vi "single path processing time test.vi"() -> ()   [LabVIEW 2010]
panel:
  out "x-y":u16
  out "updated max path lengths":u16[](array[numeric])
  in  "index":i32
  in  "Wheel Angle":i8
  in  "y LIDAR position(in)":i16
  in  "x LIDAR position(in)":i16
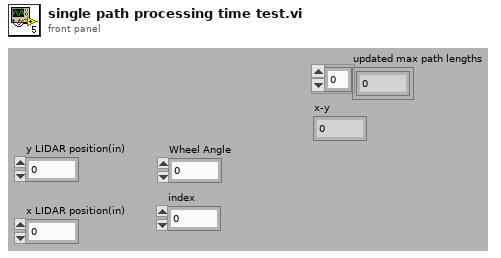
[diagram p1: front panel]
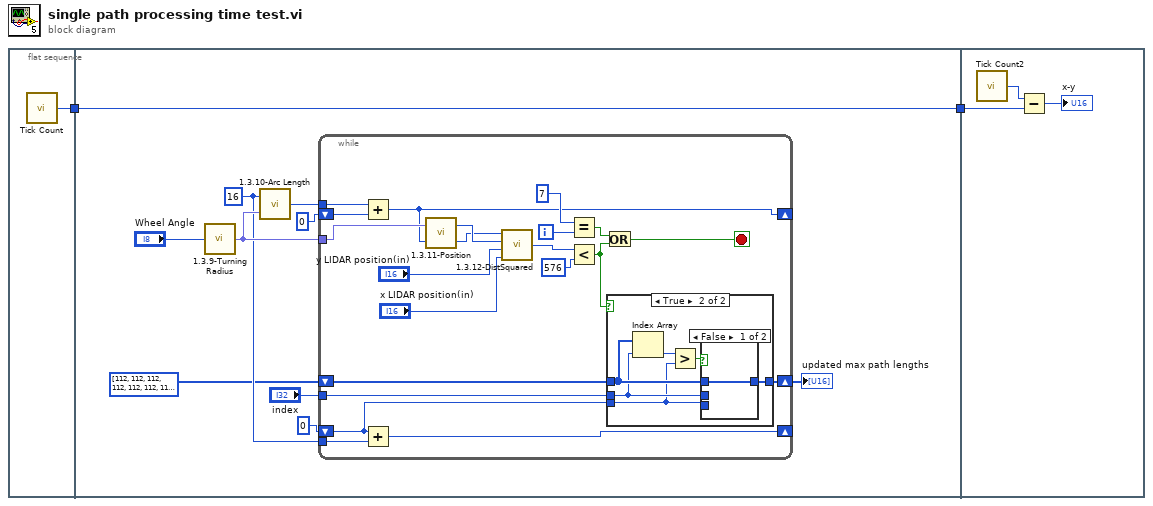
[diagram p0: block diagram]
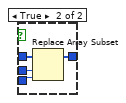
[diagram p3: hidden frame]
diagram:
  n1 = flat-sequence {
    tunnel: [w3] -> w1
    tunnel: [w4] -> w2
    tunnel: w1 -> [w4]
    tunnel: w2 -> [w49]
    frame #0 {
      n2 = call "Tick Count"() -> ("Tick Count(Ticks)"=w3:u16)
    }
    frame #1 {
      w10 = u16 16 ("Distance Along Arc")
      n3 = call "1.3.9-Turning Radius.vi"("Wheel Angle"="Wheel Angle") -> ("Turning Radius (in)"=w13:fxp<+/-,22,12>)
      n4 = call "1.3.10-Arc Length.vi"("Turning Radius (in)"=w13, "Distance Along Arc"=w10) -> ("arc length angle"=w12:u16)
      n5 = while {
        tunnel: w13 -> [w33]
        tunnel: w12 -> [w34]
        shift-right: [w17] -> _
        shift-left: u16 0 ("arc length angle") -> [w25]
        tunnel: "index" -> [w24]
        shift-right: [w23] -> w5
        shift-left: u16[] [112, 112, 112, 112, 112, 112, 112, 112, 112, 112, 112, 112, 112, 112, 112, 112] ("updated max path lengths") -> [w26]
        tunnel: w10 -> [w16]
        shift-right: [w15] -> _
        shift-left: u16 0 -> [w14]
        i -> [w22]
        stop <- w18 stop-if-true
        n6 = Add(x=w34, y=w25) -> (x+y=w17:u16)
        n7 = Add(x=w14, y=w16) -> (x+y=w15:u16)
        n8 = call "1.3.11-Position.vi"("arc length angle"=w17, "Turning Radius (in)"=w33) -> ("New Y Position"=w31:i16, "New X Position"=w32:i16)
        n9 = call "1.3.12-DistSquared.vi"("x LIDAR position"="x LIDAR position(in)", "y LIDAR position"="y LIDAR position(in)", "x position"=w32, "y position"=w31) -> ("distance squared"=w28:i16)  [unwired: 2 in]
        n10 = Equal?(x=7 ("number 16\" iterations"), y=w22) -> (x = y?=w19:bool)
        n11 = Less?(x=w28, y=576) -> (x < y?=w20:bool)
        n12 = Or(x=w19, y=w20) -> (x .or. y?=w18:bool)
        n13 = case shown="True" w20 {
          tunnel: w26 -> [w35 w40]
          tunnel: w14 -> [_ w37]
          tunnel: w24 -> [_ w39]
          tunnel: [w35 w41] -> w23
          frame False {
          }
          frame True {
            n14 = Index Array(array=w40, index=w39) -> (element=w38:u16)
            n15 = Greater?(x=w38, y=w37) -> (0:w36:bool)
            n16 = case shown="False" w36 {
              tunnel: [w42 w46] -> w41
              tunnel: w40 -> [w42 w45]
              tunnel: w39 -> [_ w44]
              tunnel: w37 -> [_ w43]
              frame False {
              }
              frame True {
                n17 = Replace Array Subset(array=w45, new element=w43, index=w44) -> (w46:u16[])
              }
            }
          }
        }
      }
      "updated max path lengths" <- w5
    }
    frame #2 {
      n18 = call "Tick Count2"() -> ("Tick Count(Ticks)"=w48:u16)
      n19 = Subtract(x=w48, y=w49) -> (x-y=→"x-y":u16)
    }
  }
